vi "BonOMM-SAOMM.Test.vi"() -> ()   [LabVIEW 2011] (continued)
                                n2786 = call "ad2xy.vi"("DEC"=w6737, "RA"=w6738, "Astrometry"=w6736) -> ("Y"=w6735:dbl, "X"=w6734:dbl)  [unwired: 6 in, 1 out]
                                n2787 = local read "Table VRN"() -> (w6731:refnum<visa-resource-name>)
                                n2788 = local read "Table Error"() -> (w6730:errorcluster)
                                n2789 = control-ref of="Table actif"() -> (w6732:refnum<vi>)
                                n2790 = call "Newmark-GotoAll.vi"("Table VRN IN"=w6731, "Bool Refnum"=w6732, "Notify?"=FALSE, "Error IN"=w6730, "Position X"=w6734, "Position Y"=w6735, "Position Z"=w6733) -> ("Table VRN OUT"=w6729:refnum<visa-resource-name>, "Error OUT"=w6728:errorcluster)  [unwired: 7 in]
                                n2791 = local write "Table Error"(w6728) -> ()
                                n2792 = local write "Table VRN"(w6729) -> ()
                                n2793 = local write "Cible X"(w6734) -> ()
                                n2794 = local write "Cible Z"(w6733) -> ()
                                n2795 = local write "Cible Y"(w6735) -> ()
                                }
                                }
                              }
                              frame True {
                                n2796 = stacked-sequence {
                                tunnel: w6767 -> [w6781 _]
                                frame #0 {
                                # "Est (180)"
                                # "Ouest (0)"
                                # "Sud (270)"
                                # "Nord (90)"
                                n2797 = case shown="2" w6781 {
                                tunnel: [45.0 90.0 270.0 180.0 0.0] -> w6780
                                frame Default {
                                }
                                frame 1 {
                                # "Nord"
                                }
                                frame 2 {
                                # "Sud"
                                }
                                frame 4 {
                                # "Est"
                                }
                                frame 8 {
                                # "Ouest"
                                }
                                }
                                n2798 = local read "RotationEffective"() -> (w6782:dbl)
                                n2799 = local read "Position X"() -> (w6779:dbl)
                                n2800 = local read "Position Y"() -> (w6778:dbl)
                                n2801 = call "FieldInterference.vi"("XCorner"=dbl[] [0.0, 500000.0, 500000.0, 0.0], "Rotation"=w6782, "YCorner"=dbl[] [0.0, 0.0, 500000.0, 500000.0], "Xsonde"=w6779, "Ysonde"=w6778, "Direction"=w6780) -> ("XCible"=w6775:dbl, "YCible"=w6774:dbl)  [unwired: 6 in, 2 out]
                                n2802 = local read "vitesse jog"() -> (w6768:dbl)
                                n2803 = local read "Table VRN"() -> (w6770:refnum<visa-resource-name>)
                                n2804 = control-ref of="Table actif"() -> (w6769:refnum<vi>)
                                n2805 = local read "Table Error"() -> (w6771:errorcluster)
                                n2806 = call "Newmark-JogLinear.vi"("Table VRN IN"=w6770, "Bool Refnum"=w6769, "Error IN"=w6771, "Position X"=w6775, "Position Y"=w6774, "Vitesse Jog"=w6768) -> ("Table VRN OUT"=w6773:refnum<visa-resource-name>, "Error OUT"=w6772:errorcluster)  [unwired: 8 in]
                                n2807 = local write "Cible X"(w6775) -> ()
                                n2808 = local write "Table VRN"(w6773) -> ()
                                n2809 = local write "Table Error"(w6772) -> ()
                                n2810 = local write "Cible Y"(w6774) -> ()
                                }
                                frame #1 {
                                n2811 = flat-sequence {
                                frame #0 {
                                n2812 = while {
                                stop <- w6795 continue-if-true
                                n2813 = local read "Exceptions"() -> (w6789:T3)
                                n2814 = local read "go Nord"() -> (w6792:bool)
                                n2815 = local read "go Ouest"() -> (w6794:bool)
                                n2816 = local read "go Est"() -> (w6793:bool)
                                n2817 = local read "go Sud"() -> (w6791:bool)
                                n2818 = Compound Arithmetic op=OR(w6794, w6793, w6792, w6791) -> (w6790:bool)
                                n2819 = Unbundle By Name(w6789) -> ("Overtravel"=w6788:bool)
                                n2820 = Not(x=w6788) -> (.not. x?=w6796:bool)
                                n2821 = Wait (ms)(milliseconds to wait=u32 50) -> ()  [unwired: 1 out]
                                n2822 = And(x=w6790, y=w6796) -> (x .and. y?=w6795:bool)
                                }
                                }
                                frame #1 {
                                n2823 = local read "Table VRN"() -> (w6808:refnum<visa-resource-name>)
                                n2824 = local read "Table Error"() -> (w6807:errorcluster)
                                n2825 = control-ref of="Table actif"() -> (w6798:refnum<vi>)
                                n2826 = local read "vitesse rapide"() -> (w6800:dbl)
                                n2827 = local read "vitesse lente"() -> (w6801:dbl)
                                n2828 = local read "accelleration"() -> (w6799:dbl)
                                n2829 = control-ref of="Table actif"() -> (w6809:refnum<vi>)
                                n2830 = call "Newmark-Stop.vi"("Table VRN IN"=w6808, "Bool Refnum"=w6809, "Error IN"=w6807) -> ("Table VRN OUT"=w6806:refnum<visa-resource-name>, "Error OUT"=w6805:errorcluster)  [unwired: 11 in]
                                n2831 = for {
                                tunnel: w6806 -> [w6818]
                                tunnel: w6805 -> [w6817]
                                tunnel: [w6816] -> w6804
                                tunnel: [w6815] -> w6803
                                tunnel: string[] ["AX", "AY"] -> [w6814] mode=indexing
                                tunnel: w6801 -> [w6813]
                                tunnel: w6800 -> [w6812]
                                tunnel: w6799 -> [w6811]
                                tunnel: w6798 -> [w6810]
                                n2832 = call "Newmark-SetSpeed.vi"("Table VRN"=w6818, "StageTAG"=w6814, "Bool Refnum"=w6810, "Error IN"=w6817, "Vitesse Lente"=w6813, "Vitesse Rapide"=w6812, "Accélération"=w6811) -> ("Table VRN OUT"=w6816:refnum<visa-resource-name>, "Error OUT"=w6815:errorcluster)  [unwired: 6 in, 1 out]
                                }
                                n2833 = local write "Table VRN"(w6804) -> ()
                                n2834 = local write "Table Error"(w6803) -> ()
                                }
                                }
                                }
                                }
                              }
                            }
                          }
                          frame #1 {
                            # "Pas certain que ce soit une\nbonne idée ... devrait être\nenvoyé en même temps <<"
                            n2835 = disable-structure shown="Disabled" {
                              frame Disabled {
                                n2836 = local write "CurvCorrect"(TRUE ("CurvCorrect")) -> ()
                              }
                              frame Enabled {
                              }
                            }
                          }
                        }
                      }
                    }
                  }
                }
              }
              event "enfoncé": Value Change {
                n2837 = event-data() -> ()  [unwired: 1 in, 6 out]
                n2838 = local read "act_cible"() -> (w6822:bool)
                n2839 = local read "act_sonde"() -> (w6821:bool)
                n2840 = Not(x=w6821) -> (.not. x?=w6824:bool)
                n2841 = Not(x=w6822) -> (.not. x?=w6823:bool)
                n2842 = local write "enfoncé"(FALSE ("enfoncé")) -> ()
                n2843 = local write "act_sonde"(w6824) -> ()
                n2844 = local write "act_cible"(w6823) -> ()
              }
              event "Obslib": Mouse Up {
                n2845 = event-data() -> ()  [unwired: 1 in, 7 out]
                n2846 = property on="Librairie des objets" class="Tbl (strict)"() -> ("Selection Start"=w6828:T43, "Selection Size"=w6827:T43)  [unwired: 2 in, 2 out]
                n2847 = Unbundle(w6828) -> ("Row"=w6844:i32)  [unwired: 1 out]
                n2848 = Unbundle(w6827) -> ("Row"=w6843:i32)  [unwired: 1 out]
                n2849 = property on="Obslib" class="Tbl (strict)"() -> ("Selection Start"=w6832:T43, "Selection Size"=w6831:T43)  [unwired: 2 in, 2 out]
                n2850 = Add(x=w6844, y=w6843) -> (x+y=w6842:i32)
                n2851 = Unbundle(w6832) -> ("Row"=w6833:i32)  [unwired: 1 out]
                n2852 = Unbundle(w6831) -> ("Row"=w6834:i32)  [unwired: 1 out]
                n2853 = Add(x=w6833, y=w6834) -> (x+y=w6835:i32)
                n2854 = Bundle(1, 9) -> (w6825:cluster{i32, i32})  [unwired: 1 in]
                n2855 = Bundle(w6842, 0) -> (w6826:cluster{i32, i32})  [unwired: 1 in]
                n2856 = property on="Librairie des objets" class="Tbl (strict)"("Selection Start"=w6826, "Selection Size"=w6825) -> ()  [unwired: 2 in, 2 out]
                n2857 = Bundle(1, 9) -> (w6829:cluster{i32, i32})  [unwired: 1 in]
                n2858 = Bundle(w6835, 0) -> (w6830:cluster{i32, i32})  [unwired: 1 in]
                n2859 = property on="Obslib" class="Tbl (strict)"("Selection Start"=w6830, "Selection Size"=w6829) -> ()  [unwired: 2 in, 2 out]
              }
              event "Reference X": Value Change {
                n2860 = event-data() -> ("OldVal"=w6849:dbl, "NewVal"=w6847:dbl)  [unwired: 1 in, 4 out]
                n2861 = In Range and Coerce(upper limit=725000, x=w6847, lower limit=575000 ("upper limit")) -> (In Range?=w6848:bool)  [unwired: 1 out]
                n2862 = case shown="False" w6848 {
                  tunnel: w6849 -> [w6850 _]
                  frame False {
                    n2863 = Two Button Dialog(message="Vous avez mis des valeurs de centres qui semble bizarres,\nVoulez-vous vraiment utiliser celles-ci comme valeurs de centres ?", 1:"NON" ("F button name (\"Cancel\")"), 2:"OUI" ("T button name (\"OK\")")) -> (T button?=w6851:bool)
                    n2864 = case shown="True" w6851 {
                      tunnel: w6850 -> [w6855 _]
                      frame False {
                        n2865 = local write "Reference X"(w6855) -> ()
                      }
                      frame True {
                        n2866 = control-ref of="TERMINAL"() -> (w6856:refnum<vi>)
                        n2867 = control-ref of="Indicateur d'état"() -> (w6857:refnum<vi>)
                        n2868 = call "TERMINAL.vi"("Indicateur Refnum"=w6857, "Terminal Refnum"=w6856, "Indicateur d'état"="Modification des valeurs en X pour le centre instrumental" ("T button name (\"OK\")")) -> ()
                      }
                    }
                  }
                  frame True {
                  }
                }
              }
              event "Reference Y": Value Change {
                n2869 = event-data() -> ("OldVal"=w6863:dbl, "NewVal"=w6861:dbl)  [unwired: 1 in, 4 out]
                n2870 = In Range and Coerce(upper limit=150000 ("lower limit"), x=w6861, lower limit=0 ("upper limit")) -> (In Range?=w6862:bool)  [unwired: 1 out]
                n2871 = case shown="False" w6862 {
                  tunnel: w6863 -> [w6864 _]
                  frame False {
                    n2872 = Two Button Dialog(message="Vous avez mis des valeurs de centres qui semble bizarres,\nVoulez-vous vraiment utiliser celles-ci comme valeurs de centres ?", 1:"NON" ("F button name (\"Cancel\")"), 2:"OUI" ("T button name (\"OK\")")) -> (T button?=w6865:bool)
                    n2873 = case shown="True" w6865 {
                      tunnel: w6864 -> [w6869 _]
                      frame False {
                        n2874 = local write "Reference Y"(w6869) -> ()
                      }
                      frame True {
                        n2875 = control-ref of="TERMINAL"() -> (w6870:refnum<vi>)
                        n2876 = control-ref of="Indicateur d'état"() -> (w6871:refnum<vi>)
                        n2877 = call "TERMINAL.vi"("Indicateur Refnum"=w6871, "Terminal Refnum"=w6870, "Indicateur d'état"="Modification des valeurs en Y pour le centre instrumental" ("T button name (\"OK\")")) -> ()
                      }
                    }
                  }
                  frame True {
                  }
                }
              }
              event "load-histo(L)": Mouse Up {
                n2878 = event-data() -> ()  [unwired: 1 in, 8 out]
                n2879 = case shown="True" "load-histo(L)" {
                  frame False {
                  }
                  frame True {
                    n2880 = local read "Librairie des objets"() -> (w6874:string[][])
                    n2881 = property on="Librairie des objets" class="Tbl (strict)"() -> ("Selection Start"=w6876:T43)  [unwired: 2 in, 2 out]
                    n2882 = local write "load-histo(L)"(FALSE ("Charger le l'objet #1")) -> ()
                    n2883 = Unbundle(w6876) -> ("Row"=w6891:i32)  [unwired: 1 out]
                    n2884 = local write "MainTab"(u32 0) -> ()
                    n2885 = Index Array(array=w6874, index (row)=w6891) -> (element=w6877:string[])  [unwired: 1 in]
                    n2886 = Index Array(array=w6877, index #1=2, index #2=3, index #3=4) -> (element #1=w6888:string, element #2=w6889:string, element #3=w6890:string)
                    n2887 = Concatenate Strings("Désirez-vous charger la coordonnées : \nRA = ", w6888, "\nDEC = ", w6889, "\nEpoch = ", w6890) -> (w6883:string)
                    n2888 = Two Button Dialog(message=w6883, 1:"NON" ("F button name (\"Cancel\")"), 2:"OUI" ("T button name (\"OK\")")) -> (T button?=w6887:bool)
                    n2889 = case shown="True" w6887 {
                      tunnel: w6888 -> [_ w6898]
                      tunnel: w6889 -> [_ w6897]
                      tunnel: w6890 -> [_ w6896]
                      tunnel: w6877 -> [_ w6895]
                      tunnel: w6877 -> [_ w6893]
                      frame False {
                      }
                      frame True {
                        n2890 = flat-sequence {
                          tunnel: w6898 -> [w6918]
                          tunnel: w6897 -> [w6917]
                          tunnel: w6896 -> [w6916]
                          tunnel: w6895 -> [w6935]
                          tunnel: [w6926] -> w6894
                          tunnel: w6894 -> [w6942]
                          tunnel: w6893 -> [w6943]
                          frame #0 {
                            w6922 = ", "
                            w6924 = 3600.0 ("y")
                            n2891 = call "time-str-to-time-dbl-RA.vi"("Chaîne"=w6918) -> ("TCS_coords"=w6903:dbl)
                            n2892 = call "time-str-to-time-dbl-DEC.vi"("Chaîne"=w6917) -> ("TCS_coords"=w6902:dbl)
                            n2893 = call "time-str-to-time-dbl.vi"("Chaîne"=w6916) -> ("TCS_coords"=w6901:dbl)
                            n2894 = local read "LST"() -> (w6913:dbl)
                            n2895 = Multiply(x=w6903, y=w6924) -> (x*y=w6915:dbl)
                            n2896 = Multiply(x=w6902, y=w6924) -> (x*y=w6914:dbl)
                            n2897 = control-ref of="TERMINAL"() -> (w6919:refnum<vi>)
                            n2898 = control-ref of="Indicateur d'état"() -> (w6920:refnum<vi>)
                            n2899 = control-ref of="TCS actif"() -> (w6899:refnum<vi>)
                            n2900 = local read "TCS VRN"() -> (w6907:refnum<visa-resource-name>)
                            n2901 = Build Array(w6903, w6902, w6901) -> (w6904:dbl[])
                            n2902 = call "Object_properties.vi"("Target RA"=w6915, "Target DEC"=w6914, "Target Epoch"=w6901, "Sideral Time"=w6913) -> ("NO RA"=w6912:string, "NO DEC"=w6911:string, "NO Epoch"=w6910:dbl, "NO HA"=w6909:dbl, "NO AM"=w6908:dbl)  [unwired: 7 in]
                            n2903 = Concatenate Strings("Chargement de l'objet : ", w6918, w6922, w6917, w6922, w6916) -> (w6923:string)
                            n2904 = call "EXCOM-CMD.vi"("VRN IN"=w6907, "Bool Refnum"=w6899, "Commande #"=6, "Args"=w6904) -> ("VRN OUT"=w6905:refnum<visa-resource-name>, "Error OUT"=w6900:errorcluster)  [unwired: 9 in, 1 out]
                            n2905 = local write "TCS Error"(w6900) -> ()
                            n2906 = call "TERMINAL.vi"("Indicateur Refnum"=w6920, "Terminal Refnum"=w6919, "Indicateur d'état"=w6923) -> ()
                            n2907 = local write "TCS VRN"(w6905) -> ()
                            n2908 = local write "NO epoch"(w6910) -> ()
                            n2909 = local write "NO AM"(w6908) -> ()
                            n2910 = local write "NO HA"(w6909) -> ()
                            n2911 = local write "N.O. Déc."(w6911) -> ()
                            n2912 = local write "N.O. A.D."(w6912) -> ()
                          }
                          frame #1 {
                            n2913 = Index Array(array=w6935, index #1=4 ("index"), index #2=5 ("index")) -> (element #1=w6931:string, element #2=w6932:string)
                            n2914 = Not Equal?(x=w6932, y="") -> (x != y?=w6928:bool)
                            n2915 = Not Equal?(x="", y=w6931) -> (x != y?=w6929:bool)
                            n2916 = local write "From library"(TRUE) -> ()
                            n2917 = Or(x=w6929, y=w6928) -> (x .or. y?=w6927:bool)
                            n2918 = case shown="True" w6927 {
                              selector: w6927 -> [w6937 _]
                              tunnel: [w6937 w6938] -> w6926
                              frame False {
                              }
                              frame True {
                                n2919 = Two Button Dialog(message="Désirez-vous également charger\nles paramètres de guidage ?  ", 1:"NON" ("F button name (\"Cancel\")"), 2:"OUI" ("T button name (\"OK\")")) -> (T button?=w6938:bool)
                              }
                            }
                          }
                          frame #2 {
                            n2920 = case shown="True" w6942 {
                              tunnel: w6943 -> [_ w6955]
                              frame False {
                              }
                              frame True {
                                w6946 = 60.0 ("x")
                                n2921 = call "Time-str-array-to-time-dbl-array.vi"("Array-str"=w6955) -> ("Array-dbl"=w6956:dbl[])
                                n2922 = Index Array(array=w6956, index #1=4, index #2=5, index #3=0 ("index"), index #4=1 ("index"), index #5=6 ("index"), index #6=7 ("index")) -> (element #1=w6960:dbl, element #2=w6958:dbl, element #3=w6959:dbl, element #4=w6957:dbl, element #5=w6952:dbl, element #6=w6951:dbl)
                                n2923 = To Single Precision Float(number=w6952) -> (single precision float=w6949:sgl)
                                n2924 = To Single Precision Float(number=w6951) -> (single precision float=w6950:sgl)
                                n2925 = local write "XReference"(w6949) -> ()
                                n2926 = local write "YReference"(w6950) -> ()
                                n2927 = Subtract(x=w6960, y=w6959) -> (x-y=w6947:dbl)
                                n2928 = Subtract(x=w6958, y=w6957) -> (x-y=w6948:dbl)
                                n2929 = Multiply(x=w6946, y=w6947) -> (x*y=w6944:dbl)
                                n2930 = Multiply(x=w6946, y=w6948) -> (x*y=w6945:dbl)
                                n2931 = property on="TableXYPos" class="XYGraph (strict)"("Cursor.Cursor Position:Cursor X"=w6944, "Cursor.Cursor Position:Cursor Y"=w6945) -> ()  [unwired: 2 in, 2 out]
                              }
                            }
                          }
                        }
                      }
                    }
                  }
                }
              }
              event "SET ZERO": Mouse Up {
                n2932 = event-data() -> ()  [unwired: 1 in, 8 out]
                n2933 = local read "MC-BonOMM VRN"() -> (w6968:refnum<visa-resource-name>)
                n2934 = call "MC-BonOMM_talker.vi"("MC-BonOMM VRN"=w6968, "Commande"="z" ("write buffer"), "Timeout (ms)"=1000, "answer=command?"=TRUE) -> ("ok ?"=w6965:bool)  [unwired: 1 in, 1 out]
                n2935 = local write "MC_connect"(w6965) -> ()
                n2936 = case shown="True" w6965 {
                  frame False {
                    n2937 = One Button Dialog(message="Erreur lors de la mise à zéro", button name ("OK")="OK ?!?") -> ()  [unwired: 1 out]
                  }
                  frame True {
                  }
                }
              }
              event "ST_RAZ": Mouse Up {
                n2938 = event-data() -> ()  [unwired: 1 in, 8 out]
                n2939 = local read "MC-BonOMM VRN"() -> (w6975:refnum<visa-resource-name>)
                n2940 = call "MC-BonOMM_talker.vi"("MC-BonOMM VRN"=w6975, "Commande"="p" ("write buffer"), "Timeout (ms)"=10000, "answer=command?"=TRUE) -> ("ok ?"=w6972:bool)  [unwired: 1 in, 1 out]
                n2941 = local write "MC_connect"(w6972) -> ()
                n2942 = case shown="False" w6972 {
                  frame False {
                    n2943 = One Button Dialog(message="Délai dépasser !?!", button name ("OK")="Heu, ok ?!?") -> ()  [unwired: 1 out]
                  }
                  frame True {
                  }
                }
              }
              event "ST_SPD": Mouse Up {
                n2944 = event-data() -> ()  [unwired: 1 in, 8 out]
                n2945 = local read "MC-BonOMM VRN"() -> (w6980:refnum<visa-resource-name>)
                n2946 = call "Change_speed.vi"("ST_SPD"="ST_SPD", "MC-BonOMM VRN"=w6980) -> ("Connected?"=w6979:bool)
                n2947 = local write "MC_connect"(w6979) -> ()
                n2948 = case shown="False" w6979 {
                  frame False {
                    n2949 = property on="Périphérique" class="Ring (strict)"("Value (Signaling)"=u16 3) -> ()  [unwired: 2 in, 2 out]
                  }
                  frame True {
                  }
                }
              }
              event "Load-library": Value Change {
                n2950 = event-data() -> ()  [unwired: 1 in, 6 out]
                n2951 = local write "Load-library"(FALSE ("Load-library")) -> ()
                n2952 = case shown="True" "Load-library" {
                  frame False {
                  }
                  frame True {
                    # "Chemin à confirmer,\nvoir avec Mr Turbide ..."
                    n2953 = local read "path_libdir"() -> (w6986:path)
                    n2954 = File Dialog(6:"*" ("pattern"), 7:"Sélectionner la libraire désirée ..." ("prompt"), 11:w6986) -> (0:w6985:errorcluster, 2:w6990:bool, 3:w6987:path)  [unwired: 4 in, 1 out]
                    n2955 = Unbundle(w6985) -> ()  [unwired: 3 out]
                    n2956 = case shown="True" w6990 {
                      tunnel: w6987 -> [_ w6992]
                      frame False {
                      }
                      frame True {
                        n2957 = local write "Load-library"(FALSE) -> ()
                        n2958 = local write "loaded_lib"(w6992) -> ()
                        n2959 = Strip Path(path=w6992) -> (stripped path=w6995:path)  [unwired: 1 out]
                        n2960 = local read "LST"() -> (w6993:dbl)
                        n2961 = call "Read_obs_files.vi"("Path"=w6992) -> ("Output Table"=w6994:string[][])  [unwired: 1 out]
                        n2962 = for {
                          tunnel: w6994 -> [w7008] mode=indexing
                          tunnel: w6993 -> [w7009]
                          tunnel: [w7005] -> w6991 mode=indexing
                          n2963 = Index Array(array=w7008, index #1=2 ("index"), index #2=3 ("index")) -> (element #1=w7011:string, element #2=w7010:string)
                          n2964 = call "Airmass.vi"("temps sidéral"=w7009, "DEC"=w7010, "RA"=w7011) -> ("airmass"=w7006:dbl)
                          n2965 = Number To Fractional String(number=w7006, precision (6)=i16 2) -> (F-format string=w7007:string)  [unwired: 2 in]
                          n2966 = Insert Into Array(array=w7008, index=5, new element=w7007) -> (w7005:string[])
                        }
                        "Librairie complète" <- w6991
                        "Librairie des objets" <- w6991
                        n2967 = Path To String(path=w6995) -> (string=w6996:string)
                        n2968 = control-ref of="TERMINAL"() -> (w7002:refnum<vi>)
                        n2969 = control-ref of="Indicateur d'état"() -> (w7001:refnum<vi>)
                        n2970 = Concatenate Strings("Chargement de la librairie \"", w6996, "\"") -> (w6999:string)
                        n2971 = call "TERMINAL.vi"("Indicateur Refnum"=w7001, "Terminal Refnum"=w7002, "Indicateur d'état"=w6999) -> ()
                      }
                    }
                  }
                }
              }
              event "modify-librairy": Value Change {
                n2972 = event-data() -> ()  [unwired: 1 in, 6 out]
                n2973 = case shown="True" "modify-librairy" {
                  frame False {
                  }
                  frame True {
                    n2974 = local read "loaded_lib"() -> (w7023:path)
                    n2975 = call "Liste-maker.vi"("Path"=w7023) -> ("Save Path"=w7016:path)
                    n2976 = local read "LST"() -> (w7024:dbl)
                    n2977 = call "Read_obs_files.vi"("Path"=w7016) -> ("path used"=w7015:path, "Output Table"=w7026:string[][])
                    n2978 = for {
                      tunnel: w7026 -> [w7032] mode=indexing
                      tunnel: w7024 -> [w7033]
                      tunnel: [w7029] -> w7025 mode=indexing
                      n2979 = Index Array(array=w7032, index #1=2 ("index"), index #2=3 ("index")) -> (element #1=w7035:string, element #2=w7034:string)
                      n2980 = call "Airmass.vi"("temps sidéral"=w7033, "DEC"=w7034, "RA"=w7035) -> ("airmass"=w7030:dbl)
                      n2981 = Number To Fractional String(number=w7030, precision (6)=i16 2) -> (F-format string=w7031:string)  [unwired: 2 in]
                      n2982 = Insert Into Array(array=w7032, index=5, new element=w7031) -> (w7029:string[])
                    }
                    n2983 = local write "loaded_lib"(w7015) -> ()
                    n2984 = Path To String(path=w7015) -> (string=w7017:string)
                    n2985 = local write "Librairie des objets"(w7025) -> ()
                    n2986 = control-ref of="TERMINAL"() -> (w7019:refnum<vi>)
                    n2987 = control-ref of="Indicateur d'état"() -> (w7018:refnum<vi>)
                    n2988 = Concatenate Strings("Modification de la librairie \"", w7017, "\"") -> (w7022:string)
                    n2989 = call "TERMINAL.vi"("Indicateur Refnum"=w7018, "Terminal Refnum"=w7019, "Indicateur d'état"=w7022) -> ()
                  }
                }
              }
              event "Rechercher...": Mouse Down {
                n2990 = event-data() -> ()  [unwired: 1 in, 8 out]
                n2991 = while {
                  stop <- w7044 continue-if-true
                  n2992 = local read "Librairie complète"() -> (w7039:string[][])
                  n2993 = local read "Rechercher..."() -> (w7042:string)
                  n2994 = call "Update_library.vi"("Librairie des objets"=w7039, "String to Search"=w7042) -> ("lib_out"=w7041:string[][])
                  n2995 = local read "Classé par ..."() -> (w7043:i32)
                  n2996 = Wait (ms)(milliseconds to wait=u32 25) -> ()  [unwired: 1 out]
                  n2997 = call "Sort_table.vi"("Column"=w7043, "Table-In"=w7041) -> ("Table-Out"=w7040:string[][])
                  n2998 = local write "Librairie des objets"(w7040) -> ()
                  n2999 = property on="Rechercher..." class="Str"() -> ("Key Focus"=w7044:bool)  [unwired: 2 in, 2 out]
                }
              }
              event "Classé par ...": Value Change {
                n3000 = event-data() -> ()  [unwired: 1 in, 6 out]
                n3001 = local read "Librairie des objets"() -> (w7047:string[][])
                n3002 = local read "Classé par ..."() -> (w7045:i32)
                n3003 = call "Sort_table.vi"("Column"=w7045, "Table-In"=w7047) -> ("Table-Out"=w7046:string[][])
                n3004 = local write "Librairie des objets"(w7046) -> ()
              }
              event "centrer_curseur_table": Value Change {
                n3005 = event-data() -> ()  [unwired: 1 in, 6 out]
                n3006 = case shown="True" "centrer_curseur_table" {
                  frame False {
                  }
                  frame True {
                    n3007 = property on="TableXYPos" class="XYGraph (strict)"("Active Cursor"=u32 1 ("Cursor.Cursor Index")) -> (error out=w7052:errorcluster, "Cursor.Cursor Position"=w7050:T44)  [unwired: 2 in, 1 out]
                    n3008 = local write "centrer_curseur_table"(FALSE) -> ()
                    n3009 = property on="TableXYPos" class="XYGraph (strict)"(error in=w7052, "Active Cursor"=u32 0 ("Cursor.Cursor Index"), "Cursor.Cursor Position"=w7050) -> ()  [unwired: 1 in, 2 out]
                  }
                }
              }
              event "centrer_curseur": Value Change {
                n3010 = event-data() -> ()  [unwired: 1 in, 6 out]
                n3011 = local write "centrer_curseur"(FALSE ("centrer_curseur")) -> ()
                n3012 = flat-sequence {
                  frame #0 {
                    n3013 = local write "CursorLock"(TRUE ("CursorLock")) -> ()
                  }
                  frame #1 {
                    n3014 = property on="TableXYPos" class="XYGraph (strict)"() -> ("XScale.Maximum"=w7063:dbl, "XScale.Minimum"=w7062:dbl)  [unwired: 2 in, 2 out]
                    n3015 = property on="TableXYPos" class="XYGraph (strict)"() -> ("YScale.Maximum"=w7059:dbl, "YScale.Minimum"=w7058:dbl)  [unwired: 2 in, 2 out]
                    n3016 = Add(x=w7063, y=w7062) -> (x+y=w7064:dbl)
                    n3017 = Add(x=w7059, y=w7058) -> (x+y=w7060:dbl)
                    n3018 = expression code="x/2"(w7064) -> (w7061:dbl)
                    n3019 = expression code="x/2"(w7060) -> (w7057:dbl)
                    n3020 = property on="TableXYPos" class="XYGraph (strict)"("Active Cursor"=u32 0, "Cursor.Cursor X"=w7061, "Cursor.Cursor Y"=w7057) -> ()  [unwired: 2 in, 2 out]
                  }
                  frame #2 {
                    n3021 = local write "CursorLock"(FALSE ("CursorLock")) -> ()
                  }
                }
              }
              event "SaveExcpt": Value Change {
                n3022 = event-data() -> ()  [unwired: 1 in, 6 out]
                n3023 = case shown="False" "SaveExcpt" {
                  frame False {
                  }
                  frame True {
                    n3024 = global read "Globals.vi" "BonOMM VI Refnum"() -> (w7073:refnum<vi>)
                    n3025 = invoke class="VI" method="Ctrl Val.Get All (Deprecated)"(reference=w7073, "controls"=FALSE) -> (reference out=w7072:refnum<vi>, error out=w7071:errorcluster, "Get All Control Values"=w7068:T45)  [unwired: 2 in, 1 out]
                    n3026 = invoke class="VI" method="Ctrl Val.Get All (Deprecated)"(reference=w7072, error in=w7071, "controls"=TRUE) -> ("Get All Control Values"=w7067:T45)  [unwired: 1 in, 3 out]
                    n3027 = call "Save_Params.vi"("Indicators"=w7068, "Controls"=w7067) -> ()  [unwired: 1 in, 1 out]
                  }
                }
              }
              event "Offset RA", "Offset DEC": Value Change; "OffRA_dir", "OffDEC_dir": Mouse Down {
                n3028 = event-data() -> ("CtlRef"=w7081:refnum<vi>)  [unwired: 1 in, 3 out]
                n3029 = property class="Ctl"(reference=w7081) -> ("Label.Text"=w7080:string)  [unwired: 1 in, 2 out]
                n3030 = local read "Offset DEC"() -> (w7078:dbl)
                n3031 = local read "Offset RA"() -> (w7079:dbl)
                n3032 = case shown="\"OffDEC_dir\"" w7080 {
                  tunnel: w7079 -> [w7083 w7084 w7088]
                  tunnel: w7078 -> [w7082 w7086 w7089]
                  tunnel: [w7083 w7084 w7087] -> w7075
                  tunnel: [w7082 w7085 w7089] -> w7074
                  frame "Offset A.D.", "Offset Déc.", Default {
                  }
                  frame "OffDEC_dir" {
                    n3033 = Negate(x=w7086) -> (-x=w7085:dbl)
                    n3034 = local write "Offset DEC"(w7085) -> ()
                    n3035 = local write "Offset RA"(w7084) -> ()
                  }
                  frame "OffRA_dir" {
                    n3036 = Negate(x=w7088) -> (-x=w7087:dbl)
                    n3037 = local write "Offset DEC"(w7089) -> ()
                    n3038 = local write "Offset RA"(w7087) -> ()
                  }
                }
                n3039 = call "Set_Offset_dir.vi"("DEC"=w7074, "RA"=w7075) -> ("DEC_dir"=→"OffDEC_dir":string, "RA_dir"=→"OffRA_dir":string)
              }
              event "Offset RA", "Offset DEC": Mouse Down {
                n3040 = event-data() -> ()  [unwired: 1 in, 8 out]
              }
              event "copy_calib", "copy_ref", "copy_centre": Value Change {
                n3041 = event-data() -> ("CtlRef"=w7098:refnum<vi>)  [unwired: 1 in, 5 out]
                n3042 = property class="Bool"(reference=w7098) -> ("Label.Text"=w7097:string)  [unwired: 1 in, 2 out]
                n3043 = case shown="\"copy_ref\"" w7097 {
                  tunnel: ["<NO REFERENCE>" "de calibration" "de la référence instrumentale" "du centre optique"] -> w7093
                  frame Default {
                  }
                  frame "copy_calib" {
                  }
                  frame "copy_ref" {
                  }
                  frame "copy_centre" {
                  }
                }
                n3044 = Concatenate Strings("Êtes vous certain de vouloir modifier la position ", w7093, " ?") -> (w7092:string)
                n3045 = Two Button Dialog(message=w7092, 1:"NON" ("T button name (\"OK\")"), 2:"OUI" ("T button name (\"OK\")")) -> (T button?=w7096:bool)
                n3046 = case shown="True" w7096 {
                  tunnel: w7097 -> [_ w7099]
                  frame False {
                  }
                  frame True {
                    n3047 = local read "Position X"() -> (w7102:dbl)
                    n3048 = local read "Position Y"() -> (w7101:dbl)
                    n3049 = local read "Position Z"() -> (w7100:dbl)
                    n3050 = case shown="\"copy_centre\"" w7099 {
                      tunnel: w7102 -> [_ w7104 w7106 w7108]
                      tunnel: w7101 -> [_ w7103 w7105 w7107]
                      tunnel: w7100 -> [_ _ _ _]
                      frame Default {
                      }
                      frame "copy_calib" {
                        n3051 = local write "Calibration X"(w7104) -> ()
                        n3052 = local write "Calibration Y"(w7103) -> ()
                      }
                      frame "copy_ref" {
                        n3053 = local write "Reference X"(w7106) -> ()
                        n3054 = local write "Reference Y"(w7105) -> ()
                      }
                      frame "copy_centre" {
                        n3055 = local write "CentreTel X"(w7108) -> ()
                        n3056 = local write "CentreTel Y"(w7107) -> ()
                      }
                    }
                  }
                }
              }
              event "Cen-Snd-RA", "Cen-Snd-DEC", "Cen-Cib-RA", "Cen-Cib-DEC": Value Change {
                n3057 = event-data() -> ()  [unwired: 1 in, 6 out]
                n3058 = disable-structure shown="Disabled" {
                  frame Disabled {
                    n3059 = local read "Cen-Snd-DEC"() -> ()  [unwired: 1 out]
                    n3060 = local read "Cen-Snd-RA"() -> ()  [unwired: 1 out]
                  }
                  frame Enabled {
                  }
                }
                n3061 = call "format_string2arcmin.vi"("Arcmin-Str"="Cen-Cib-DEC") -> ("Arcmin"=w7116:dbl)  [unwired: 14 in]
                n3062 = call "format_string2arcmin.vi"("Arcmin-Str"="Cen-Cib-RA") -> ("Arcmin"=w7117:dbl)  [unwired: 14 in]
                n3063 = property on="TableXYPos" class="XYGraph (strict)"("Active Cursor"=u32 0, "Cursor.Cursor X"=w7117, "Cursor.Cursor Y"=w7116) -> ()  [unwired: 2 in, 2 out]
              }
              event "best_target": Value Change {
                # "Remettre les conditions sur BestTargetLed"
                n3064 = event-data() -> ()  [unwired: 1 in, 6 out]
                n3065 = stacked-sequence {
                  frame #0 {
                    n3066 = local write "best_target"(FALSE ("best_target")) -> ()
                    n3067 = property on="best_target" class="Bool (strict)"("DisabledEnum"=T17."Disabled" ("Disabled")) -> ()  [unwired: 2 in, 2 out]
                  }
                  frame #1 {
                    # "Vérifie si le data est à date ..."
                    n3068 = local read "BestTargetLed"() -> (w7120:bool)
                    n3069 = case shown="False" w7120 {
                      frame False {
                        n3070 = local read "DEC-Champ"() -> (w7122:dbl)
                        n3071 = local read "RA-Champ"() -> (w7123:dbl)
                        n3072 = local write "BestTargetLed"(FALSE ("BestTargetLed")) -> ()
                        n3073 = flat-sequence {
                          tunnel: [w7132] -> w7124
                          tunnel: w7123 -> [w7129]
                          tunnel: w7122 -> [w7128]
                          tunnel: w7124 -> [w7150]
                          frame #0 {
                            # "R1mag limite USNO"
                            n3074 = local read "Représentation"() -> (w7127:dbl)
                            n3075 = local read "path_data"() -> (w7134:path)
                            n3076 = local read "wgetexec"() -> (w7133:path)
                            n3077 = Add(x=w7127, y=10.0) -> (x+y=w7125:dbl)
                            n3078 = while {
                              stop <- w7138 stop-if-true
                              n3079 = local read "BestTargetLed"() -> (w7140:bool)
                              n3080 = Wait (ms)(milliseconds to wait=u32 333) -> ()  [unwired: 1 out]
                              n3081 = Not(x=w7140) -> (.not. x?=w7139:bool)
                              n3082 = local write "BestTargetLed"(w7139) -> ()
                              n3083 = local read "USNO_ready"() -> (w7138:bool)
                            }
                            n3084 = call "QueryUSNO.vi"("wget"=w7133, "Data dir Path"=w7134, "mag_limit"=12.0, "radius"=w7125, "DEC"=w7128, "RA"=w7129) -> ("Data OUT"=w7135:string[][], "No Error"=w7130:bool)  [unwired: 3 in, 1 out]
                            n3085 = case shown="True" w7130 {
                              tunnel: w7135 -> [_ w7149]
                              tunnel: w7130 -> [w7142 w7147]
                              tunnel: [w7142 w7147] -> w7132
                              tunnel: [TRUE TRUE] -> w7131
                              tunnel: w7129 -> [_ w7144]
                              tunnel: w7128 -> [_ w7143]
                              frame False {
                              }
                              frame True {
                                # "6 = R1mag"
                                n3086 = call "Sort_USNO_data.vi"("Column Used"=6, "Data IN"=w7149) -> ("Data OUT"=w7145:string[][])  [unwired: 8 in, 1 out]
                                n3087 = local write "USNO_data"(w7145) -> ()
                                "RA-USNO" <- w7144
                                "DEC-USNO" <- w7143
                              }
                            }
                            n3088 = local write "USNO_ready"(w7131) -> ()
                          }
                          frame #1 {
                            n3089 = local write "USNO_ready"(w7150) -> ()
                            "BestTargetLed" <- w7150
                          }
                        }
                      }
                      frame True {
                      }
                    }
                  }
                  frame #2 {
                    n3090 = local read "BestTargetLed"() -> (w7151:bool)
                    n3091 = case shown="True" w7151 {
                      frame False {
                      }
                      frame True {
                        w7152 = u16 1 items=["Region d'intérêt", "Prévisualisation", "Idle"] ("ImageUsage")
                        # "Proper motion limit (mas/yr)"
                        # "Pickup mirror footprint (arcmin)"
                        # "R1mag lower limit"
                        n3092 = local read "FOV"() -> (w7180:dbl)
                        n3093 = local read "TableAstrom"() -> (w7163:T4)
                        n3094 = local read "USNO_data"() -> (w7185:string[][])
                        n3095 = local read "Epoch Tel"() -> (w7182:dbl)
                        n3096 = local read "DEC Tel"() -> (w7183:dbl)
                        n3097 = local read "RA Tel"() -> (w7184:dbl)
                        n3098 = call "Choose_best_target(multi).vi"("R1mag lower limit"=6.0, "FOV"=w7180, "Footprint"=1.0, "PM limit"=25.0 ("Footprint"), "EPOCH TEL"=w7182, "DEC TEL"=w7183, "Table Astrometry"=w7163, "RA TEL"=w7184, "USNO_data"=w7185) -> ("Best Target"=w7162:string[][], "target RA (deg)"=w7171:dbl, "target DEC (deg)"=w7170:dbl)  [unwired: 3 in, 5 out]
                        "Target Data" <- w7162
                        n3099 = local read "FirstBest"() -> (w7169:bool)
                        n3100 = case shown="False" w7169 {
                          selector: w7169 -> [_ w7203]
                          tunnel: w7171 -> [_ w7205]
                          tunnel: [w7189 w7205] -> w7159
                          tunnel: w7170 -> [_ w7204]
                          tunnel: [w7188 w7204] -> w7158
                          tunnel: w7162 -> [w7200 _]
                          frame False {
                            n3101 = Increment(x="BestCount") -> (x+1=w7196:i32)
                            n3102 = Index Array(array=w7200, index (row)="BestCount") -> (element=w7197:string[])  [unwired: 1 in]
                            n3103 = Quotient & Remainder(x=w7196, y=3) -> (x-y*floor(x/y)=w7199:i32)  [unwired: 1 out]
                            n3104 = Index Array(array=w7197) -> (element #1=w7195:string, element #2=w7194:string, element #3=w7193:string)  [unwired: 3 in]
                            n3105 = local read "Epoch Tel"() -> (w7186:dbl)
                            n3106 = Fract/Exp String To Number(string=w7195) -> (number=w7192:dbl)  [unwired: 3 in, 1 out]
                            n3107 = Fract/Exp String To Number(string=w7194) -> (number=w7191:dbl)  [unwired: 3 in, 1 out]
                            n3108 = Fract/Exp String To Number(string=w7193) -> (number=w7190:dbl)  [unwired: 3 in, 1 out]
                            n3109 = local write "BestCount"(w7199) -> ()
                            n3110 = call "precess.vi"("Eq2"=w7186, "Eq1"=w7190, "DEC 1"=w7191, "RA 1"=w7192) -> ("DEC 2"=w7188:dbl, "RA 2"=w7189:dbl)
                          }
                          frame True {
                            n3111 = Not(x=w7203) -> (.not. x?=→"FirstBest":bool)
                            n3112 = local write "BestCount"(1 ("BestCount")) -> ()
                          }
                        }
                        n3113 = local read "ImageDSSLed"() -> (w7172:bool)
                        n3114 = local read "Epoch Tel"() -> (w7156:dbl)
                        n3115 = call "precess.vi"("Eq2"=2000.0, "Eq1"=w7156, "DEC 1"=w7158, "RA 1"=w7159) -> ("DEC 2"=w7154:dbl, "RA 2"=w7155:dbl)
                        n3116 = call "deg2ad.vi"("DEC (°)"=w7158, "RA (°)"=w7159) -> ("DEC (°)"=→"RA-USNO-sec 3":dbl, "RA (sec)"=→"RA-USNO-sec 2":dbl)
                        n3117 = case shown="False" w7172 {
                          tunnel: w7155 -> [w7210 w7229]
                          tunnel: w7154 -> [w7209 w7228]
                          tunnel: [w7207 w7227] -> w7174
                          frame False {
                            w7211 = 2.0 ("Size")
                            n3118 = local read "wgetexec"() -> (w7213:path)
                            n3119 = local read "path_dss"() -> (w7212:path)
                            n3120 = call "Query_Vizier.vi"("Folder"=w7212, "wget"=w7213, "Width"=w7211, "Height"=w7211, "DEC"=w7209, "RA"=w7210) -> ("error?"=w7206:bool, "Path2Image"=w7208:path)  [unwired: 4 in]
                            n3121 = case shown="False" w7206 {
                              tunnel: w7208 -> [w7218 _]
                              tunnel: [w7217 w7225] -> w7207
                              frame False {
                                n3122 = call "gfitsio-open-create-replace-file.vi"("file path (dialog if empty)"=w7218) -> ("error out"=w7223:errorcluster, "gfits refnum"=w7222:T46)  [unwired: 8 in, 1 out]
                                n3123 = call "gfitsio-read-header.vi"("error in (no error)"=w7223, "gfits refnum"=w7222) -> ("error out"=w7220:errorcluster, "dup gfits refnum"=w7221:T46)  [unwired: 7 in, 1 out]
                                n3124 = call-poly "gfitsio-read-image-subset.vi"("lpixel (-1,-1: rest)"=cluster{"X":i32, "Y":i32} {"X"=-1, "Y"=-1}, "fpixel (1,1)"=cluster{"X":i32, "Y":i32} {"X"=1, "Y"=1}, "error in (no error)"=w7220, "gfits refnum"=w7221) -> ("error out"=w7216:errorcluster, "data"=w7217:sgl[][], "dup gfits refnum"=w7215:T46)  [unwired: 4 in, 1 out]
                                n3125 = call "gfitsio-close-file.vi"("error in (no error)"=w7216, "gfits refnum"=w7215) -> ("error out"=→"fits Error":errorcluster)  [unwired: 8 in, 1 out]
                              }
                              frame True {
                                w7226 = sgl 0.0 ("element")
                                n3126 = Initialize Array(w7226, w7226, w7226) -> (w7225:sgl[][])
                              }
                            }
                          }
                          frame True {
                            n3127 = local read "ImgAstrom"() -> (w7237:T4)
                            n3128 = call "ad2xy.vi"("DEC"=w7228, "RA"=w7229, "Astrometry"=w7237) -> ("Y"=w7234:dbl, "X"=w7235:dbl)  [unwired: 6 in, 1 out]
                            n3129 = To Long Integer(number=w7235) -> (32bit integer=w7233:i32)
                            n3130 = To Long Integer(number=w7234) -> (32bit integer=w7232:i32)
                            n3131 = local read "ImgData"() -> (w7236:sgl[][])
                            n3132 = call "subimage.vi"("Ysz/2"=100, "Xsz/2"=100, "Yc"=w7232, "Xc"=w7233, "ImgData"=w7236) -> ("SubImg"=w7227:sgl[][])  [unwired: 6 in]
                          }
                        }
                        n3133 = local read "FieldAstrom"() -> (w7176:T4)
                        n3134 = local write "SubIMG4DSS?"(TRUE ("SubIMG4DSS?")) -> ()
                        n3135 = call "ad2xy.vi"("DEC"=w7158, "RA"=w7159, "Astrometry"=w7176) -> ("Y"=w7164:dbl, "X"=w7165:dbl)  [unwired: 6 in, 1 out]
                        n3136 = property on="TableXYPos" class="XYGraph (strict)"("Active Cursor"=u32 0, "Cursor.Cursor Position:Cursor X"=w7165, "Cursor.Cursor Position:Cursor Y"=w7164) -> ()  [unwired: 2 in, 2 out]
                        n3137 = call "format_arcmin2arcsecstr.vi"("RA arcmin"=w7165, "DEC Arcmin"=w7164) -> ("Formatted RA"=w7168:string, "Formatted Dist"=w7166:string, "Formatted DEC"=w7167:string)  [unwired: 11 in]
                        n3138 = Array Max & Min(array=w7174) -> (max value=w7175:sgl)  [unwired: 3 out]
                        n3139 = call "Draw_crosshair.vi"("Image IN"=w7174, "White Value"=w7175) -> ("Image OUT"=w7173:sgl[][])  [unwired: 13 in]
                        n3140 = local write "Cen-Cib-TOT"(w7166) -> ()
                        n3141 = local write "Cen-Cib-RA"(w7168) -> ()
                        n3142 = local write "Cen-Cib-DEC"(w7167) -> ()
                        n3143 = local write "ImageUsage"(w7152) -> ()
                        n3144 = local write "subimg"(w7173) -> ()
                      }
                    }
                  }
                  frame #3 {
                    n3145 = property on="best_target" class="Bool (strict)"("DisabledEnum"=T17."Enabled" ("Disabled")) -> ()  [unwired: 2 in, 2 out]
                  }
                }
              }
              event "GetDSS", "DS9": Value Change {
                # "Trace l'image DSS par dessus le champ des tables de guidage"
                n3146 = event-data() -> ("CtlRef"=w7243:refnum<vi>)  [unwired: 1 in, 4 out]
                n3147 = flat-sequence {
                  tunnel: w7243 -> [w7249]
                  tunnel: [w7248] -> w7242
                  tunnel: [w7277] -> w7245
                  tunnel: w7242 -> [w7271]
                  tunnel: [w7265] -> w7241
                  tunnel: [w7264] -> w7240
                  tunnel: [w7263] -> w7239
                  tunnel: w7245 -> [w7334]
                  tunnel: path "C:/BonOMM/BonOMM-2012/Apps/SAOImage-DS9/ds9.exe" ("DS9path") -> [w7333]
                  tunnel: w7241 -> [w7329]
                  tunnel: w7240 -> [w7331]
                  tunnel: w7239 -> [w7330]
                  frame #0 {
                    w7247 = T17."Disabled" ("Disabled")
                    w7246 = FALSE ("DSS_ready")
                    n3148 = property class="Bool (strict)"(reference=w7249) -> ("Label.Text"=w7248:string)  [unwired: 1 in, 2 out]
                    n3149 = local write "ImageDSSLed"(w7246) -> ()
                    n3150 = local write "DS9-Led"(w7246) -> ()
                    n3151 = local write "DSS_ready"(w7246) -> ()
                    n3152 = local write "DS9_ready"(w7246) -> ()
                    n3153 = local write "GetDSS"(w7246) -> ()
                    n3154 = property on="DS9" class="Bool (strict)"("DisabledEnum"=w7247) -> ()  [unwired: 2 in, 2 out]
                    n3155 = property on="GetDSS" class="Bool (strict)"("DisabledEnum"=w7247) -> ()  [unwired: 2 in, 2 out]
                    n3156 = local write "DS9"(w7246) -> ()
                  }
                  frame #1 {
                    w7296 = u16 0 items=["Square", "Circle"] ("Ring")
                    # "Invert X"
                    # "Époque DSS et USNO"
                    n3157 = local read "Reference Y"() -> (w7298:dbl)
                    n3158 = local read "Reference X"() -> (w7297:dbl)
                    n3159 = local read "CentreTel X"() -> (w7261:dbl)
                    n3160 = local read "CentreTel Y"() -> (w7260:dbl)
                    n3161 = local read "RotationEffective"() -> (w7257:dbl)
                    n3162 = local read "arcsec/pulse"() -> (w7294:dbl)
                    n3163 = local read "Représentation"() -> (w7270:dbl)
                    n3164 = To Double Precision Float(number=w7297) -> (double precision float=w7289:dbl)
                    n3165 = To Double Precision Float(number=w7298) -> (double precision float=w7288:dbl)
                    n3166 = Equal?(x=w7271, y="DS9") -> (x = y?=w7265:bool)
                    n3167 = Select(t=60.0, s=w7265, f=w7270) -> (s? t:f=w7269:dbl)
                    n3168 = local read "DEC Tel"() -> (w7291:dbl)
                    n3169 = local read "RA Tel"() -> (w7290:dbl)
                    n3170 = while {
                      tunnel: w7271 -> [w7299]
                      stop <- w7301 stop-if-true
                      n3171 = case shown="\"DS9\"" w7299 {
                        tunnel: [TRUE ("DSS_ready") w7305 "DS9_ready"] -> w7301
                        frame "False", Default {
                        }
                        frame "GetDSS" {
                          n3172 = local read "ImageDSSLed"() -> (w7303:bool)
                          n3173 = local read "DSS_ready"() -> (w7305:bool)
                          n3174 = Not(x=w7303) -> (.not. x?=→"ImageDSSLed":bool)
                        }
                        frame "DS9" {
                          n3175 = local read "DS9-Led"() -> (w7307:bool)
                          n3176 = Not(x=w7307) -> (.not. x?=→"DS9-Led":bool)
                        }
                      }
                      n3177 = Wait (ms)(milliseconds to wait=u32 333) -> ()  [unwired: 1 out]
                    }
                    n3178 = call "Set_field_astrometry.vi"("Cen x (pas)"=w7261, "effective rotation (°)"=w7257, "scale (\"/pas)"=w7294, "NaxisMax"=500000, "Cen y (pas)"=w7260, "Use Center?"=FALSE ("Ues Constant Size ?"), "Ref x (pas)"=w7289, "Ref y (pas)"=w7288, "RA (HH:MM:SS.S)"=w7290, "DEC(DD:MM:SS)"=w7291, "Inversion Cluster"=T20 {"Invert Angle"=FALSE, "Invert X"=TRUE, "Invert Y"=FALSE}) -> ("Field Astrometry"=w7283:T4, "Table Astrometry"=w7284:T4)  [unwired: 3 in]
                    n3179 = property on="TableXYPos" class="XYGraph (strict)"("Active Cursor"=u32 1) -> ("Cursor.Cursor X"=w7252:dbl, "Cursor.Cursor Y"=w7253:dbl)  [unwired: 2 in, 2 out]
                    n3180 = local read "MirVig"() -> (w7254:dbl)
                    n3181 = local read "Miroir"() -> (w7251:dbl)
                    n3182 = local read "FOV"() -> (w7295:dbl)
                    n3183 = local write "TableAstrom"(w7284) -> ()
                    n3184 = local read "NaxisMax"() -> (w7262:dbl)
                    n3185 = Bundle("Miroir"=w7251, "Cursor.Cursor X"=w7252, "Cursor.Cursor Y"=w7253, "MirVig"=w7254) -> (w7250:T47)  [unwired: 1 in]
                    n3186 = local read "Epoch Tel"() -> (w7281:dbl)
                    n3187 = call "draw_field.vi"("Field_Astrometry"=w7283, "FOV"=w7295, "NaxisMax"=w7262, "Ring"=w7296, "Table_Astrometry"=w7284, "Ues Constant Size ?"=TRUE, "margin/size"=w7269, "MirrorAvatar"=w7250) -> ("X Scale.Range"=w7276:T26, "ImgDEC"=w7256:dbl, "ImgRA"=w7280:dbl, "Y Scale.Range"=w7275:T26)  [unwired: 3 in, 1 out]
                    n3188 = call "precess.vi"("Eq2"=2000.0, "Eq1"=w7281, "DEC 1"=w7256, "RA 1"=w7280) -> ("DEC 2"=w7278:dbl, "RA 2"=w7279:dbl)
                    n3189 = local read "path_dss"() -> (w7286:path)
                    n3190 = Add(x=w7269, y=4.0) -> (x+y=w7274:dbl)
                    n3191 = local read "wgetexec"() -> (w7285:path)
                    n3192 = local write "FieldAstrom"(w7283) -> ()
                    n3193 = call "Query_Vizier.vi"("Folder"=w7286, "wget"=w7285, "Width"=w7274, "Height"=w7274, "DEC"=w7278, "RA"=w7279) -> ("error?"=w7266:bool, "Path2Image"=w7287:path)  [unwired: 4 in]
                    n3194 = local write "Img DEC"(w7278) -> ()
                    n3195 = local write "Img RA"(w7279) -> ()
                    n3196 = Or(x=w7266, y=w7265) -> (x .or. y?=w7267:bool)
                    n3197 = case shown="False" w7267 {
                      tunnel: w7279 -> [w7321 _]
                      tunnel: w7278 -> [w7320 _]
                      tunnel: w7287 -> [w7312 w7327]
                      tunnel: w7283 -> [w7318 _]
                      tunnel: [TRUE TRUE] -> w7264
                      tunnel: [w7312 w7327] -> w7277
                      tunnel: w7276 -> [w7311 _]
                      tunnel: w7275 -> [w7310 _]
                      tunnel: [w7309 FALSE] -> w7263
                      frame False {
                        # "ImgData et ImgAstrom\nsont lié à plus grand que le\nchamp affiché."
                        n3198 = property on="TableXYPos" class="XYGraph (strict)"() -> ("Height"=w7325:u32, "Width"=w7324:u32)  [unwired: 2 in, 2 out]
                        n3199 = To Long Integer(number=w7325) -> (32bit integer=w7323:i32)
                        n3200 = To Long Integer(number=w7324) -> (32bit integer=w7322:i32)
                        n3201 = call "Draw_graph_background.vi"("Y Scale.Range"=w7310, "ImgRA"=w7321, "X Scale.Range"=w7311, "ImgDEC"=w7320, "Field Astrometry"=w7318, "New Width"=w7322, "New Height"=w7323, "path"=w7312) -> ("ImgData"=w7313:sgl[][], "Astrometry"=w7317:T4, "error out"=w7315:errorcluster, "Images"=w7319:picture)
                        "DSS Error" <- w7315
                        n3202 = Unbundle By Name(w7315) -> ("status"=w7314:bool)
                        n3203 = property on="TableXYPos" class="XYGraph (strict)"("PlotImages.Back"=w7319) -> ()  [unwired: 2 in, 2 out]
                        n3204 = local write "ImgAstrom"(w7317) -> ()
                        n3205 = local write "ImgData"(w7313) -> ()
                        n3206 = Not(x=w7314) -> (.not. x?=w7309:bool)
                      }
                      frame True {
                      }
                    }
                    n3207 = local write "DSS_ready"(w7264) -> ()
                    n3208 = local write "DS9_ready"(w7264) -> ()
                  }
                  frame #2 {
                    w7332 = T17."Enabled" ("Disabled")
                    n3209 = property on="GetDSS" class="Bool (strict)"("DisabledEnum"=w7332) -> ()  [unwired: 2 in, 2 out]
                    n3210 = case shown="True" w7329 {
                      tunnel: w7334 -> [_ w7338]
                      tunnel: w7333 -> [_ w7337]
                      tunnel: w7331 -> [_ w7336]
                      tunnel: w7330 -> [w7335 _]
                      frame False {
                        n3211 = local write "ImageDSSLed"(w7335) -> ()
                      }
                      frame True {
                        n3212 = local write "DS9-Led"(w7336) -> ()
                        n3213 = call "fits2ds9.vi"("DS9path"=w7337, "FitsFile"=w7338) -> ()  [unwired: 10 in]
                      }
                    }
                    n3214 = property on="DS9" class="Bool (strict)"("DisabledEnum"=w7332) -> ()  [unwired: 2 in, 2 out]
                  }
                }
              }
              event "LVDT-Set-ZERO": Value Change {
                n3215 = event-data() -> ()  [unwired: 1 in, 5 out]
                n3216 = local write "LVDT-Set-ZERO"(FALSE ("LVDT-Set-ZERO")) -> ()
                n3217 = flat-sequence {
                  tunnel: [w7343] -> w7339
                  tunnel: w7339 -> [w7344]
                  frame #0 {
                    n3218 = Two Button Dialog(message="Assurez-vous que les moteurs sont éteints depuis au\nmoins 30 secondes et que les plateaux sont bien engagés.", 1:"Annuler" ("F button name (\"Cancel\")")) -> (T button?=w7343:bool)  [unwired: 1 in]
                  }
                  frame #1 {
                    n3219 = case shown="True" w7344 {
                      frame False {
                      }
                      frame True {
                        n3220 = local read "Graph Data"() -> (w7345:dbl[])
                        n3221 = call <vilib>:"Mean.vi"("X"=w7345) -> ("mean"=w7346:dbl)  [unwired: 1 out]
                        n3222 = local write "LVDT-zero"(w7346) -> ()
                      }
                    }
                  }
                }
              }
              event "LVDT-Save-Data": Value Change {
                n3223 = event-data() -> ()  [unwired: 1 in, 5 out]
                n3224 = local write "LVDT-Save-Data"(FALSE ("want seconds? (F)")) -> ()
                n3225 = local read "LVDT-RA-Data"() -> (w7372:dbl[])
                n3226 = local read "Q String"() -> (w7368:string)
